vi "DSP_EnableFFT.vi"(2 "error in (no error)":errorcluster, 3 "Enable FFT":bool, 4 "Board Handle":u64) -> (0 "error out":errorcluster, 1 "Board Handle Out":u64)   [LabVIEW 2009]
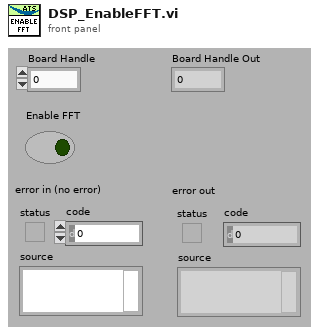
[diagram p1: front panel]
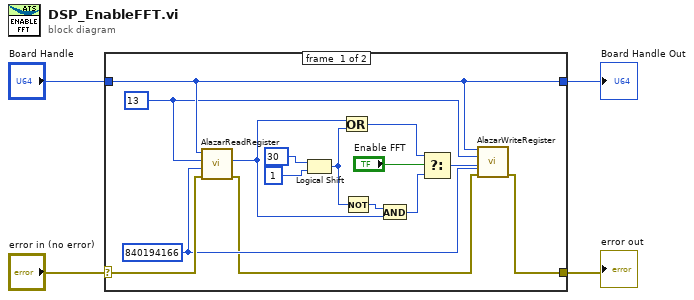
[diagram p0: block diagram]
diagram:
  n1 = case shown="No Error" "error in (no error)" {
    selector: "error in (no error)" -> [w19 w21]
    tunnel: [w5 w21] -> w3
    tunnel: [w10 w20] -> w2
    tunnel: "Board Handle" -> [w10 w20]
    frame #0 {
      w9 = u32 13
      w7 = u32 840194166
      n2 = call "AlazarReadRegister.vi"("error in (no error)"=w19, "Password"=w7, "Offset"=w9, "Board Handle"=w10) -> ("error out"=w6:errorcluster, "Value Out"=w13:u32)  [unwired: 2 out]
      n3 = Logical Shift(y=30, x=u32 1) -> (x << y=w15:u32)
      n4 = Or(x=w13, y=w15) -> (x .or. y?=w11:u32)
      n5 = Not(x=w15) -> (.not. x?=w14:u32)
      n6 = And(x=w14, y=w13) -> (x .and. y?=w12:u32)
      n7 = Select(t=w11, s="Enable FFT", f=w12) -> (s? t:f=w8:u32)
      n8 = call "AlazarWriteRegister.vi"("Board Handle"=w10, "Offset"=w9, "Value"=w8, "Password"=w7, "error in (no error)"=w6) -> ("error out"=w5:errorcluster)  [unwired: 8 in, 2 out]
    }
    frame #1 {
    }
  }
  "Board Handle Out" <- w2
  "error out" <- w3
